vi "Get_PascalCaseName.vi"(8 "error in (no error)":errorcluster, 10 "LV2011Compatibility":bool, 11 "Name":string) -> (0 "error out":errorcluster, 3 "PascalCaseName":string)   [LabVIEW 2020]
uses:
  e:/builds/penguin/labview/branches/2020/dev/dist/resource/NationalInstruments.LabVIEW.Generator.dll
  resource/NationalInstruments.LabVIEW.Generator.dll
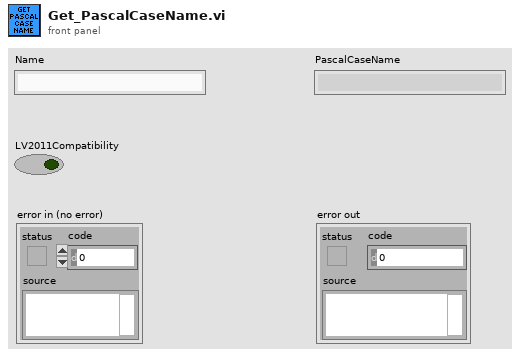
[diagram p1: front panel]
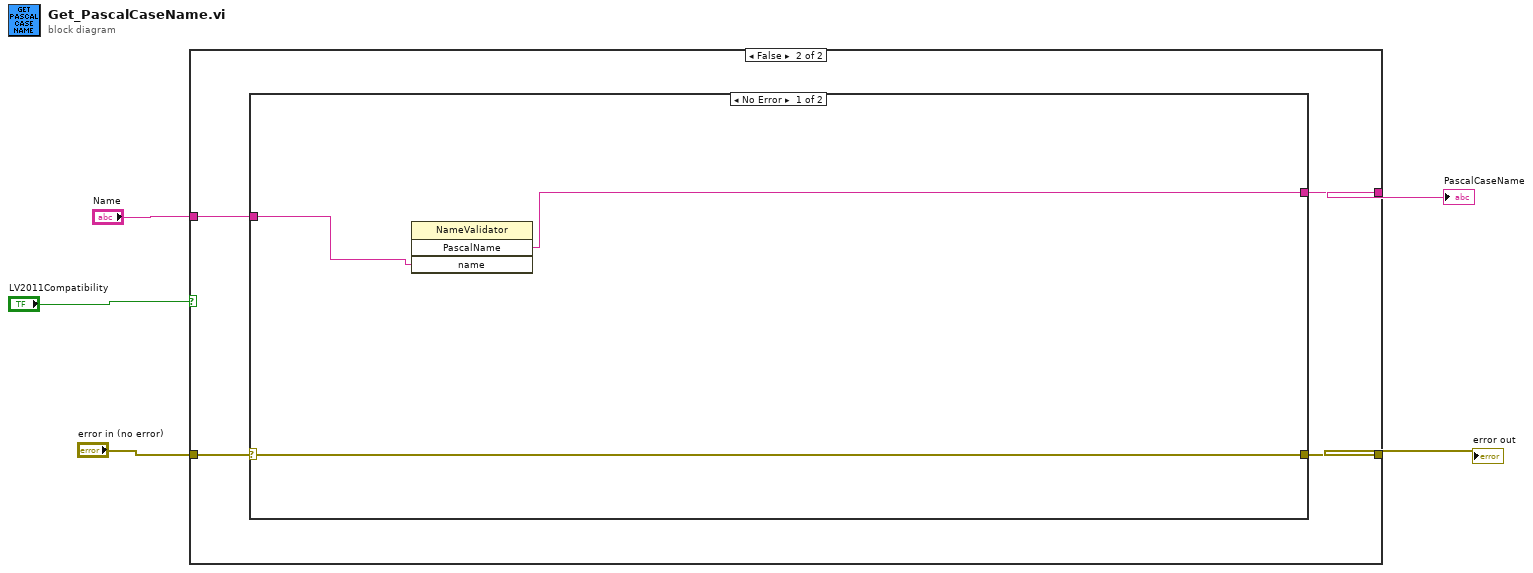
[diagram p0: block diagram]
diagram:
  n1 = case shown="False" "LV2011Compatibility" {
    tunnel: "error in (no error)" -> [w6 w11]
    tunnel: "Name" -> [w7 w10]
    tunnel: [w6 w9] -> w3
    tunnel: [w7 w8] -> w2
    frame True {
    }
    frame False {
      n2 = case shown="No Error" w11 {
        selector: w11 -> [w14 w15]
        tunnel: w10 -> [w13 _]
        tunnel: [w14 w15] -> w9
        tunnel: [w12 _] -> w8
        frame No Error {
          n3 = invoke class="NameValidator" method="PascalName"("name"=w13) -> ("PascalName"=w12:string)  [unwired: 3 in, 3 out]
        }
        frame Error {
        }
      }
    }
  }
  "PascalCaseName" <- w2
  "error out" <- w3
